vi "kr_pn.vi"(5 "Dev_Gr":cluster{"DevNo":i32, "Group":string}[](array[cluster])) -> (0 "KR":string, 1 "x = y?":bool, 2 "PN":string, 3 "Array":i32[](array[numeric]))   [LabVIEW 2010]
uses:
  Global 2.vi
panel:
  # "Первый столбец из таблицы каналов\nпереписывается как есть, из второго - только \nотсутствующие в первом!"
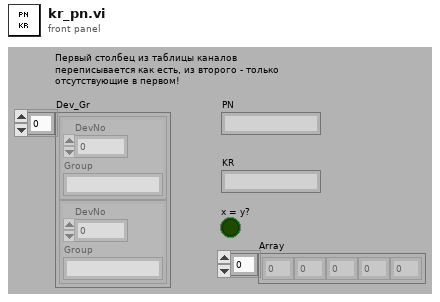
[diagram p1: front panel]
types:
  T1 = cluster{"name":enum16{"sync", "phase_a", "phase_b", "phase_c", "ground"}, "num":i32, "Numeric":i32}[]
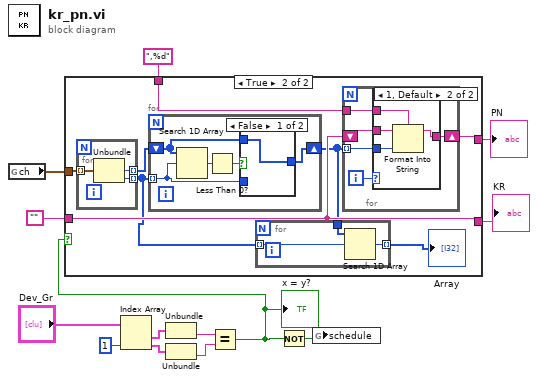
[diagram p0: block diagram]
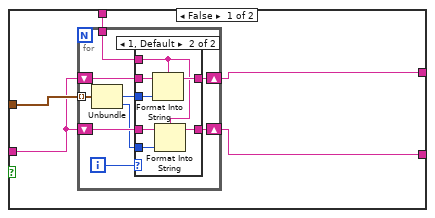
[diagram p2: hidden frame]
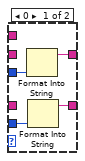
[diagram p3: hidden frame]
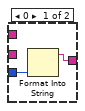
[diagram p4: hidden frame]
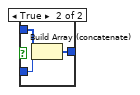
[diagram p5: hidden frame]
diagram:
  n1 = global read "Global 2.vi" "ch"() -> (w6:T1)
  n2 = Index Array(array="Dev_Gr", index #2=1 ("index")) -> (element #1=w9:cluster{"DevNo":i32, "Group":string}, element #2=w10:cluster{"DevNo":i32, "Group":string})  [unwired: 1 in]
  n3 = Unbundle(w9) -> ("Group"=w12:string)  [unwired: 1 out]
  n4 = Unbundle(w10) -> ("Group"=w11:string)  [unwired: 1 out]
  n5 = Equal?(x=w12, y=w11) -> (x = y?=w2:bool)
  "x = y?" <- w2
  n6 = case shown="True" w2 {
    tunnel: w6 -> [w18 w46]
    tunnel: [w17 w42] -> w5
    tunnel: [w16 w43] -> w4
    tunnel: "" -> [w15 w43]
    tunnel: ",%d" -> [w14 w44]
    frame False {
      n7 = for {
        shift-right: [w25] -> w17
        shift-left: w15 -> [w24]
        tunnel: w18 -> [w27] mode=indexing
        shift-right: [w21] -> w16
        shift-left: w15 -> [w22]
        tunnel: w14 -> [w19]
        i -> [w23]
        n8 = Unbundle(w27) -> ("num"=w26:i32, "Numeric"=w20:i32)  [unwired: 1 out]
        n9 = case shown="1, Default" w23 {
          tunnel: w26 -> [w31 w38]
          tunnel: [w30 w37] -> w25
          tunnel: w24 -> [_ w36]
          tunnel: w19 -> [_ w32]
          tunnel: w22 -> [_ w35]
          tunnel: [w28 w34] -> w21
          tunnel: w20 -> [w29 w33]
          frame 0 {
            n10 = Format Into String(w31) -> (resulting string=w30:string)  [unwired: 3 in, 1 out]
            n11 = Format Into String(w29) -> (resulting string=w28:string)  [unwired: 3 in, 1 out]
          }
          frame 1, Default {
            n12 = Format Into String(format string=w32, initial string=w36, w38) -> (resulting string=w37:string)  [unwired: 1 in, 1 out]
            n13 = Format Into String(format string=w32, initial string=w35, w33) -> (resulting string=w34:string)  [unwired: 1 in, 1 out]
          }
        }
      }
    }
    frame True {
      n14 = for {
        tunnel: w46 -> [w72] mode=indexing
        tunnel: [w71] -> w40 mode=indexing
        tunnel: [w70] -> w45 mode=indexing
        n15 = Unbundle(w72) -> ("num"=w70:i32, "Numeric"=w71:i32)  [unwired: 1 out]
      }
      n16 = for {
        tunnel: w40 -> [w63] mode=indexing
        shift-right: [w61] -> w41
        shift-left: w45 -> [w62]
        n17 = Search 1D Array(1D array=w62, element=w63) -> (index of element=w65:i32)  [unwired: 1 in]
        n18 = Less Than 0?(x=w65) -> (x < 0?=w64:bool)
        n19 = case shown="False" w64 {
          tunnel: w63 -> [_ w69]
          tunnel: w62 -> [w66 w68]
          tunnel: [w66 w67] -> w61
          frame False {
          }
          frame True {
            n20 = Build Array (concatenate)(w68, w69) -> (w67:i32[])
          }
        }
      }
      n21 = for {
        tunnel: w41 -> [w49]
        tunnel: w40 -> [w48] mode=indexing
        tunnel: [w47] -> w39 mode=indexing
        n22 = Search 1D Array(1D array=w49, element=w48) -> (index of element=w47:i32)  [unwired: 1 in]
      }
      "Array" <- w39
      n23 = for {
        tunnel: w41 -> [w53] mode=indexing
        tunnel: w44 -> [w52]
        shift-right: [w50] -> w42
        shift-left: w43 -> [w51]
        i -> [w54]
        n24 = case shown="1, Default" w54 {
          tunnel: w53 -> [w56 w60]
          tunnel: w52 -> [_ w59]
          tunnel: w51 -> [_ w58]
          tunnel: [w55 w57] -> w50
          frame 0 {
            n25 = Format Into String(w56) -> (resulting string=w55:string)  [unwired: 3 in, 1 out]
          }
          frame 1, Default {
            n26 = Format Into String(format string=w59, initial string=w58, w60) -> (resulting string=w57:string)  [unwired: 1 in, 1 out]
          }
        }
      }
    }
  }
  "PN" <- w5
  "KR" <- w4
  n27 = Not(x=w2) -> (.not. x?=w13:bool)
  n28 = global write "Global 2.vi" "schedule"(w13) -> ()
